vi "niRFUtil MT UTIL Decimate.vi"(0 "Signal In":T1 format="%.2f", 5 "Samples Per Symbol (16)":i32=16, 7 "Offset":i32, 11 "error in (no error)":errorcluster) -> (4 "Signal Out":T1 format="%.2f", 15 "error out":errorcluster)   [LabVIEW 2015, in "niRFUtil.lvlib"]
uses:
  niRFUtil.lvlib
  Includes/niRFUtil INC Complex Array.ctl
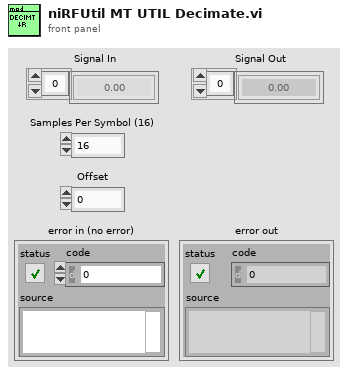
[diagram p1: front panel]
types:
  T1 = typedef "niRFUtil.lvlib/niRFUtil INC Complex Array.ctl" = csg[]
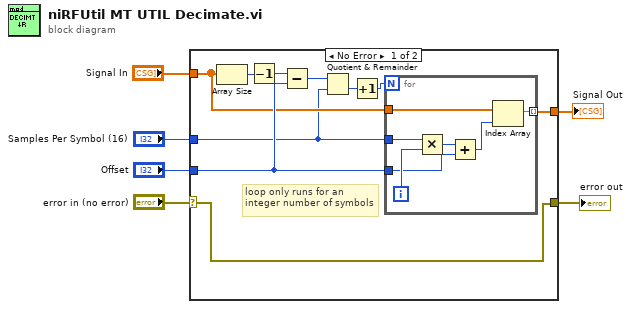
[diagram p0: block diagram]
diagram:
  n1 = case shown="No Error" "error in (no error)" {
    selector: "error in (no error)" -> [w7 w24]
    tunnel: "Signal In" -> [w14 _]
    tunnel: "Samples Per Symbol (16)" -> [w10 _]
    tunnel: "Offset" -> [w16 _]
    tunnel: [w15 _] -> w3
    tunnel: [w7 w24] -> w1
    frame No Error {
      # "loop only runs for an integer number of symbols"
      n2 = Array Size(array=w14) -> (size(s)=w13:i32)
      n3 = Decrement(x=w13) -> (x-1=w12:i32)
      n4 = Subtract(x=w12, y=w16) -> (x-y=w11:i32)
      n5 = Quotient & Remainder(x=w11, y=w10) -> (floor(x/y)=w9:i32)  [unwired: 1 out]
      n6 = Increment(x=w9) -> (x+1=w8:i32)
      n7 = for {
        N: w8 -> [_]
        tunnel: w14 -> [w23]
        tunnel: w10 -> [w22]
        tunnel: w16 -> [w19]
        tunnel: [w17] -> w15 mode=indexing
        i -> [w21]
        n8 = Multiply(x=w22, y=w21) -> (x*y=w20:i32)
        n9 = Add(x=w20, y=w19) -> (x+y=w18:i32)
        n10 = Index Array(array=w23, index=w18) -> (element=w17:csg)
      }
    }
    frame Error {
    }
  }
  "error out" <- w1
  "Signal Out" <- w3
